vi "DELETE.vi"(6 "timeout":i32=10000, 7 "output file":path, 8 "error in":errorcluster, 10 "url":string, 11 "session in":refnum<class "Session.lvclass">) -> (0 "error out":errorcluster, 1 "body":string, 2 "headers":string, 3 "Session out":refnum<class "Session.lvclass">, 4 "status code":u32)   [LabVIEW 2019, in "NI_Advanced HTTP Client.lvlib" / "Session.lvclass"]
doc: "Sends a web request to delete resources on a server, web page, or web service. This VI uses the DELETE HTTP method. The server accepting the request from the DELETE VI must be set up to delete resources solely based upon receiving a DELETE web request at the specified URL."
uses:
  Session.lvclass
  Session.lvclass/Session.ctl
  lvwebclient_32.dll
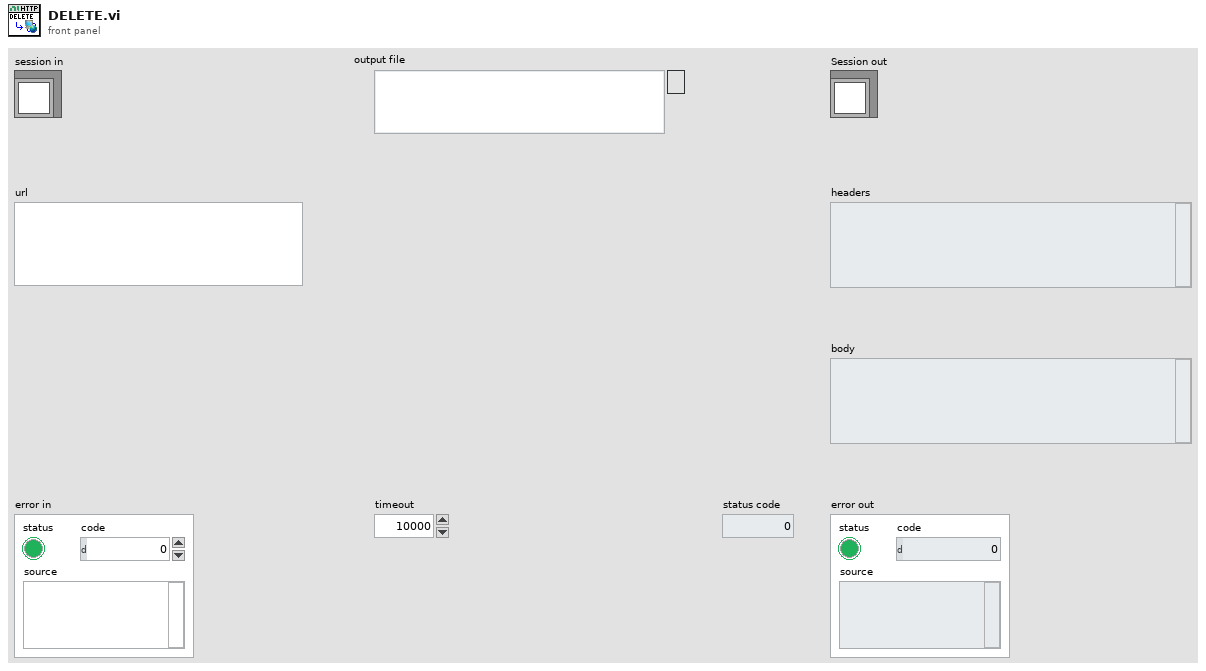
[diagram p1: front panel]
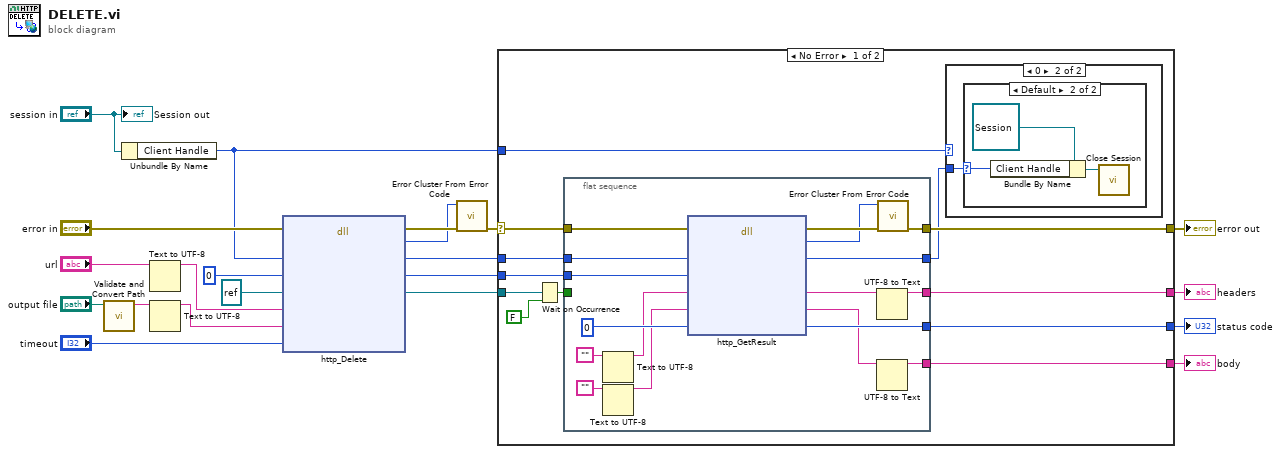
[diagram p0: block diagram]
diagram:
  n1 = call "Validate and Convert Path.vi"("path"="output file") -> ("validated path as string"=w17:string)  [unwired: 10 in]
  n2 = Unbundle By Name("session in") -> ("Client Handle"=w9:u32)
  n3 = Text to UTF-8(11:"url") -> (3:w6:string)  [unwired: 2 in, 1 out]
  n4 = Text to UTF-8(11:w17) -> (3:w5:string)  [unwired: 2 in, 1 out]
  n5 = dll-call lib="C:/source/github/ni-adv-http-api/Advanced HTTP Client/lvwebclient_*.*" fn="http_Delete"(error in="error in", "handle"=w9, "request"=u32 0, "completeOccurrence"=refnum<k4> refnum ("occurrence"), "url"=w6, "outPath"=w5, "timeout"="timeout") -> (error out=w11:errorcluster, "return"=w10:i32, "handle"=w3:u32, "request"=w2:u32, "completeOccurrence"=w1:refnum<k4>)  [unwired: 5 in, 1 out]
  n6 = call <vilib>:"Error Cluster From Error Code.vi"("error in (no error)"=w11, "error code (0)"=w10) -> ("error out"=w21:errorcluster)  [unwired: 7 in]
  n7 = case shown="No Error" w21 {
    selector: w21 -> [w31 w55]
    tunnel: w1 -> [w33 _]
    tunnel: w3 -> [w30 _]
    tunnel: w2 -> [w29 _]
    tunnel: [w28 _] -> w16
    tunnel: [w27 _] -> w15
    tunnel: [w26 _] -> w14
    tunnel: [w25 w55] -> w13
    tunnel: w9 -> [w24 _]
    frame No Error {
      n8 = Wait on Occurrence(1:FALSE, 2:w33) -> (0:w32:bool)  [unwired: 1 in]
      n9 = flat-sequence {
        tunnel: w32 -> [_]
        tunnel: w31 -> [w54]
        tunnel: w30 -> [w53]
        tunnel: w29 -> [w52]
        tunnel: [w50] -> w28
        tunnel: [w45] -> w27
        tunnel: [w44] -> w26
        tunnel: [w43] -> w25
        tunnel: [w42] -> w23
        frame #0 {
          n10 = Text to UTF-8(11:"") -> (3:w39:string)  [unwired: 2 in, 1 out]
          n11 = Text to UTF-8(11:"") -> (3:w38:string)  [unwired: 2 in, 1 out]
          n12 = dll-call lib="C:/source/github/ni-adv-http-api/Advanced HTTP Client/lvwebclient_*.*" fn="http_GetResult"(error in=w54, "handle"=w53, "request"=w52, "returnHeader"=w39, "returnBody"=w38, "httpStatus"=u32 0) -> (error out=w49:errorcluster, "return"=w48:i32, "handle"=w42:u32, "returnHeader"=w47:string, "returnBody"=w46:string, "httpStatus"=w50:u32)  [unwired: 3 in, 1 out]
          n13 = UTF-8 to Text(11:w47) -> (3:w45:string)  [unwired: 2 in, 1 out]
          n14 = UTF-8 to Text(11:w46) -> (3:w44:string)  [unwired: 2 in, 1 out]
          n15 = call <vilib>:"Error Cluster From Error Code.vi"("error in (no error)"=w49, "error code (0)"=w48) -> ("error out"=w43:errorcluster)  [unwired: 7 in]
        }
      }
      n16 = case shown="0" w24 {
        tunnel: w23 -> [_ w34]
        frame Default {
        }
        frame 0 {
          n17 = case shown="Default" w34 {
            selector: w34 -> [_ w37]
            frame 0 {
            }
            frame Default {
              n18 = Bundle By Name(cluster=refnum<class "Session.lvclass"> refnum ("NI_Advanced HTTP Client.lvlib:Session.lvclass"), "Client Handle"=w37) -> (w36:refnum<class "Session.lvclass">)
              n19 = call "Close Session.vi"("session"=w36) -> ()  [unwired: 10 in, 1 out]
            }
          }
        }
      }
    }
    frame Error {
    }
  }
  "error out" <- w13
  "headers" <- w15
  "body" <- w14
  "status code" <- w16
  "Session out" <- "session in"
